vi "4Pi 4Pi Modes - DM AE.vi"(0 "DM Handles":T1(array[cluster]), 3 "Flats":dbl[](array[numeric]), 4 "Control Matrix":dbl[][](array[numeric]), 5 "Serials":string[](array[string]), 6 "Action":T2, 7 "No hardware":bool=TRUE) -> (11 "Serials Out":string[](array[string]), 13 "No hardware Out":bool, 14 "DM Handles Out":T1(array[cluster]), 17 "Flats Out":dbl[](array[numeric]), 19 "Control Matrix Out":dbl[][](array[numeric]))   [LabVIEW 2016]
uses:
  4Pi 4Pi Modes - Controls/4Pi 4Pi Modes - Standard Action.ctl
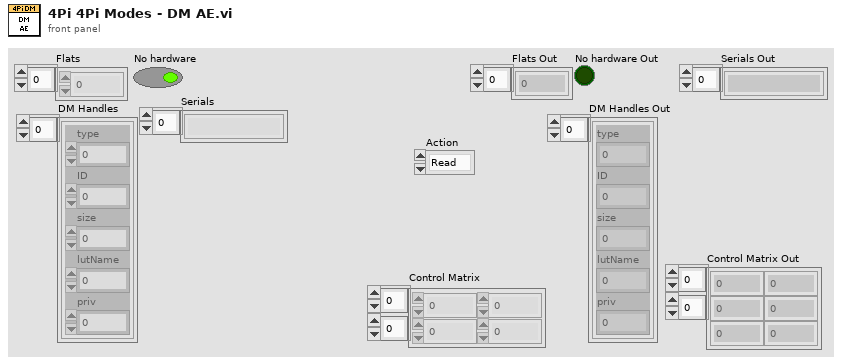
[diagram p1: front panel]
types:
  T1 = cluster{"type":i16, "ID":i16, "size":i32, "lutName":u64, "priv":u64}[]
  T2 = typedef "4Pi 4Pi Modes - Standard Action.ctl" = enum16{"Read", "Write"}
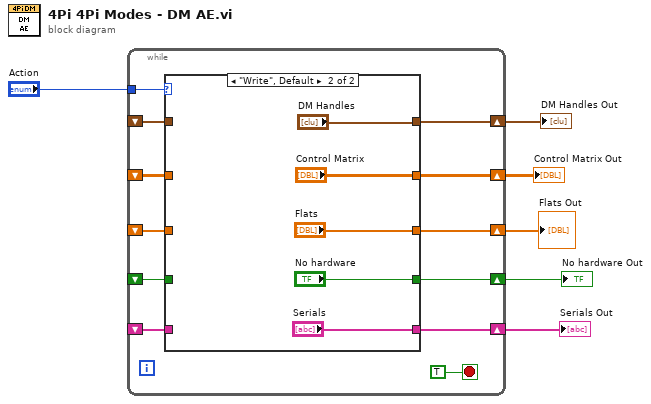
[diagram p0: block diagram]
diagram:
  n1 = while {
    tunnel: "Action" -> [w17]
    shift-right: [w13] -> w4
    shift-left: _ -> [w16]
    shift-right: [w15] -> w5
    shift-left: _ -> [w14]
    shift-right: [w12] -> w3
    shift-left: _ -> [w11]
    shift-right: [w10] -> w2
    shift-left: _ -> [w9]
    shift-right: [w8] -> w1
    shift-left: _ -> [w7]
    stop <- TRUE stop-if-true
    n2 = case shown="\"Write\", Default" w17 {
      tunnel: w16 -> [w22 _]
      tunnel: [w23 "Control Matrix"] -> w15
      tunnel: w14 -> [w23 _]
      tunnel: [w22 "Flats"] -> w13
      tunnel: [w21 "DM Handles"] -> w12
      tunnel: w11 -> [w21 _]
      tunnel: [w20 "No hardware"] -> w10
      tunnel: w9 -> [w20 _]
      tunnel: [w19 "Serials"] -> w8
      tunnel: w7 -> [w19 _]
      frame "Read" {
      }
      frame "Write", Default {
      }
    }
  }
  "Control Matrix Out" <- w5
  "Flats Out" <- w4
  "DM Handles Out" <- w3
  "No hardware Out" <- w2
  "Serials Out" <- w1
